vi "Modbus Status ES.vi"(0 "InterfaceData":T3 {"GenEast"."TotalFuel(L)" format="%.2f"; "GenEast"."FuelRate(L/H)" format="%.2f"; "GenEast"."ApparentPower(VA)" format="%.2f"; "GenEast"."BattVoltage(V)" format="%.2f"; "GenEast"."Freq(Hz)" format="%.2f"; "GenEast"."RunHours(hr)" format="%.2f"; "GenEast"."PowerFactor" format="%.2f"; "GenEast"."ReactivePower(VAR)" format="%.2f"; "GenEast"."ActivePower(W)" format="%.2f"; "GenWest"."TotalFuel(L)" format="%.2f"; "GenWest"."FuelRate(L/H)" format="%.2f"; "GenWest"."ApparentPower(VA)" format="%.2f"; "GenWest"."BattVoltage(V)" format="%.2f"; "GenWest"."Freq(Hz)" format="%.2f"; "GenWest"."RunHours(hr)" format="%.2f"; "GenWest"."PowerFactor" format="%.2f"; "GenWest"."ReactivePower(VAR)" format="%.2f"; "GenWest"."ActivePower(W)" format="%.2f"; "Converter Alarms 2" format="%016b"; "Converter Faults 2" format="%016b"; "Controller Faults" format="%016b"; "System Status" format="%016b"; "Converter Alarms 1" format="%016b"; "Converter Faults 1" format="%016b"; "Solar Faults" format="%016b"; "ES Rack 10 Alarms" format="%016b"; "ES Rack 9 Alarms" format="%016b"; "ES Rack 8 Alarms" format="%016b"; "ES Rack 7 Alarms" format="%016b"; "ES Rack 6 Alarms" format="%016b"; "ES Rack 5 Alarms" format="%016b"; "ES Rack 4 Alarms" format="%016b"; "ES Rack 3 Alarms" format="%016b"; "ES Rack 2 Alarms" format="%016b"; "ES Rack 1 Alarms" format="%016b"; "ES System Alarms" format="%016b"; "System Faults" format="%016b"; "ES Rack 10 Faults" format="%016b"; "ES Rack 9 Faults" format="%016b"; "ES Rack 8 Faults" format="%016b"; "ES Rack 7  Faults" format="%016b"; "ES Rack 6 Faults" format="%016b"; "ES Rack 5 Faults" format="%016b"; "ES Rack 4 Faults" format="%016b"; "ES Rack 3 Faults" format="%016b"; "ES Rack 2 Faults" format="%016b"; "ES Rack 1 Faults" format="%016b"; "ES System Faults" format="%016b"}, 1 "ES Cycle Count":dbl, 5 "ES String Data":T1, 9 "ES System Data In":T5={"Voltage"=0.0, "Current"=0.0, "SOC Avg"=0.0, "Faults"=0, "Alarms"=0, "# Strings"=0, "Max Temp"=0, "Min Temp"=0, "Max Cell Voltage"=0.0, "Min Cell Voltage"=0.0, "Energy Capacity"=0.0, "Energy Remaining"=0.0, "SOC Min"=0.0, "SOC Max"=0.0, "ES Fault"=FALSE, "String Select"=enum."3 Strings", "ES Com Fault"=FALSE, "SOH Avg"=0.0}, 11 "Error In":errorcluster) -> (4 "InterfaceData":T3 {"GenEast"."TotalFuel(L)" format="%.2f"; "GenEast"."FuelRate(L/H)" format="%.2f"; "GenEast"."ApparentPower(VA)" format="%.2f"; "GenEast"."BattVoltage(V)" format="%.2f"; "GenEast"."Freq(Hz)" format="%.2f"; "GenEast"."RunHours(hr)" format="%.2f"; "GenEast"."PowerFactor" format="%.2f"; "GenEast"."ReactivePower(VAR)" format="%.2f"; "GenEast"."ActivePower(W)" format="%.2f"; "GenWest"."TotalFuel(L)" format="%.2f"; "GenWest"."FuelRate(L/H)" format="%.2f"; "GenWest"."ApparentPower(VA)" format="%.2f"; "GenWest"."BattVoltage(V)" format="%.2f"; "GenWest"."Freq(Hz)" format="%.2f"; "GenWest"."RunHours(hr)" format="%.2f"; "GenWest"."PowerFactor" format="%.2f"; "GenWest"."ReactivePower(VAR)" format="%.2f"; "GenWest"."ActivePower(W)" format="%.2f"; "Converter Alarms 2" format="%016b"; "Converter Faults 2" format="%016b"; "Controller Faults" format="%016b"; "System Status" format="%016b"; "Converter Alarms 1" format="%016b"; "Converter Faults 1" format="%016b"; "Solar Faults" format="%016b"; "ES Rack 10 Alarms" format="%016b"; "ES Rack 9 Alarms" format="%016b"; "ES Rack 8 Alarms" format="%016b"; "ES Rack 7 Alarms" format="%016b"; "ES Rack 6 Alarms" format="%016b"; "ES Rack 5 Alarms" format="%016b"; "ES Rack 4 Alarms" format="%016b"; "ES Rack 3 Alarms" format="%016b"; "ES Rack 2 Alarms" format="%016b"; "ES Rack 1 Alarms" format="%016b"; "ES System Alarms" format="%016b"; "System Faults" format="%016b"; "ES Rack 10 Faults" format="%016b"; "ES Rack 9 Faults" format="%016b"; "ES Rack 8 Faults" format="%016b"; "ES Rack 7  Faults" format="%016b"; "ES Rack 6 Faults" format="%016b"; "ES Rack 5 Faults" format="%016b"; "ES Rack 4 Faults" format="%016b"; "ES Rack 3 Faults" format="%016b"; "ES Rack 2 Faults" format="%016b"; "ES Rack 1 Faults" format="%016b"; "ES System Faults" format="%016b"}, 15 "Error Out":errorcluster)   [LabVIEW 2014]
uses:
  Controls/ES System Data.ctl
  Controls/StringSelector.ctl
  Controls/Interface Data.ctl
  Controls/Gen Data.ctl
  Controls/ES String Array.ctl
  Controls/ES String Data.ctl
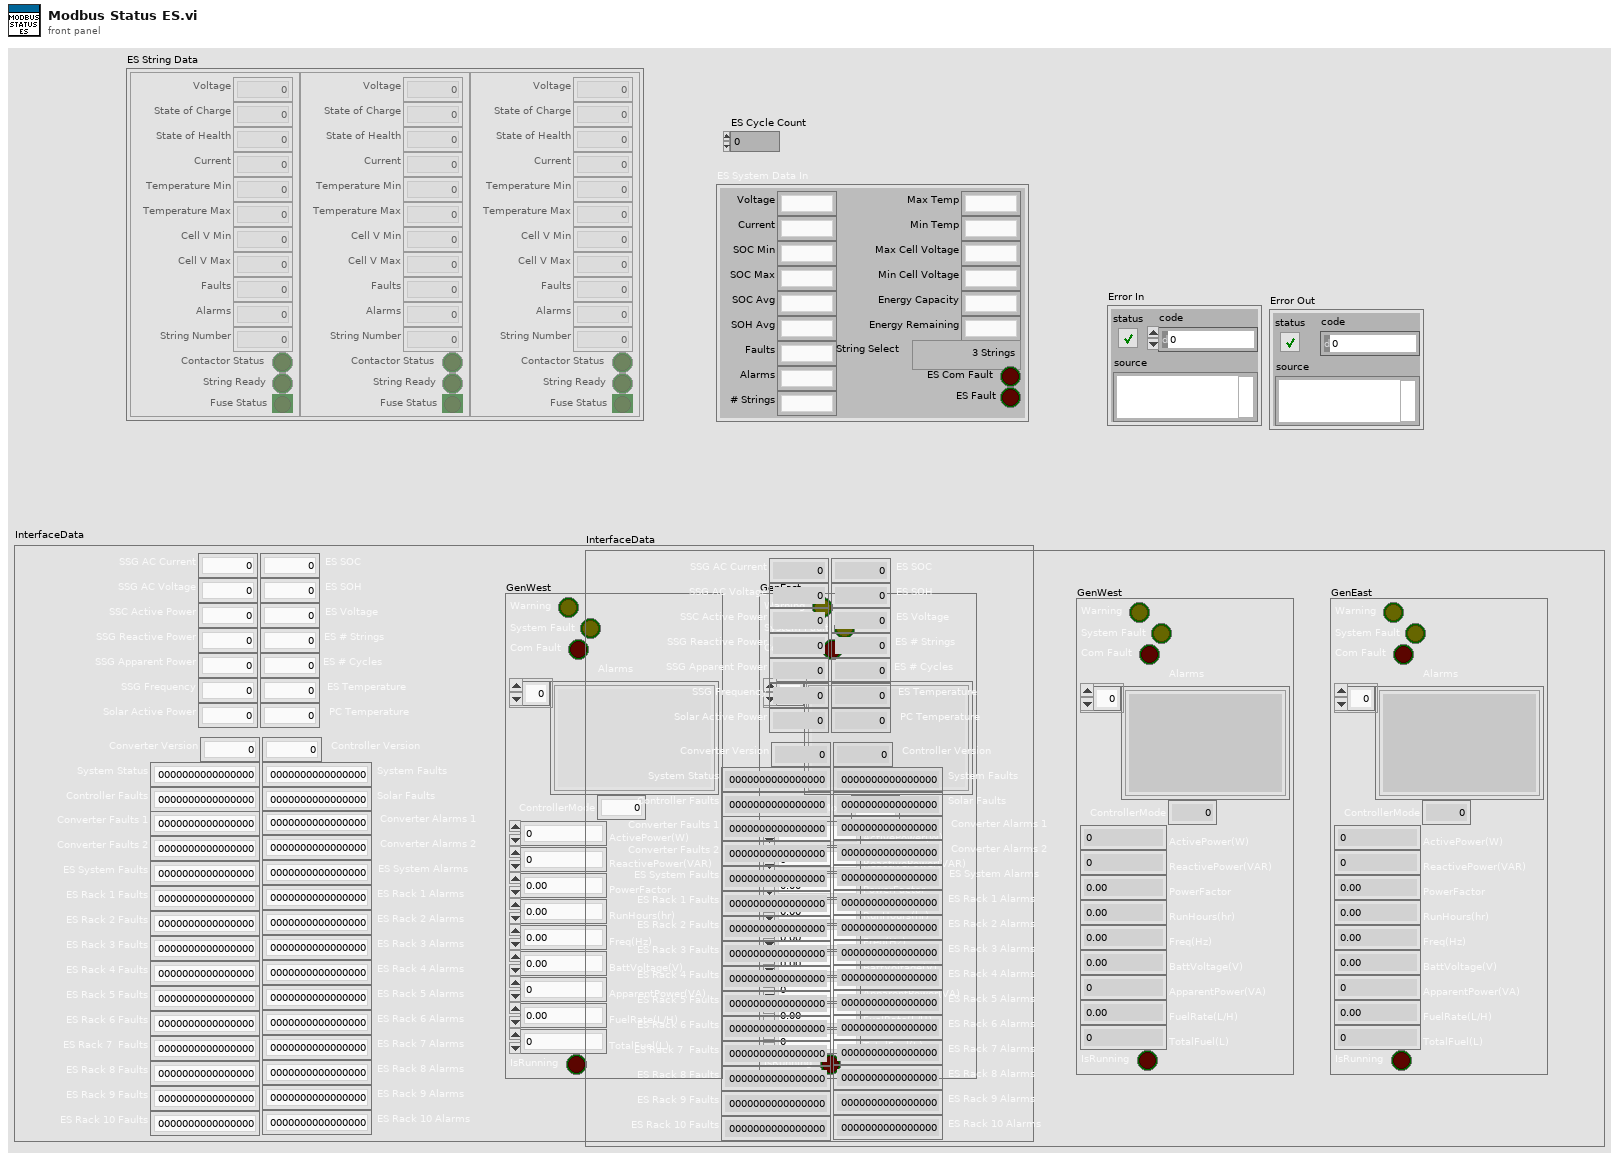
[diagram p1: front panel]
types:
  T1 = typedef "ES String Array.ctl" = T2[]
  T2 = typedef "ES String Data.ctl" = cluster{"Voltage":sgl, "State of Charge":sgl, "Current":sgl, "Temperature Min":i16, "Temperature Max":i16, "Faults":u16, "Alarms":u16, "String Number":u16, "Contactor Status":bool, "String Ready":bool, "Fuse Status":bool, "Cell V Max":dbl, "Cell V Min":dbl, "State of Health":sgl}
  T3 = typedef "Interface Data.ctl" = cluster{"SSG AC Current":i16, "SSG AC Voltage":i16, "SSC Active Power":i16, "SSG Reactive Power":i16, "SSG Apparent Power":i16, "SSG Frequency":i16, "ES SOC":i16, "ES SOH":i16, "ES Voltage":i16, "ES # Strings":i16, "ES # Cycles":i16, "ES Temperature":i16, "PC Temperature":i16, "Solar Active Power":i16, "Converter Version":i16, "Controller Version":i16, "System Status":i16, "System Faults":i16, "Controller Faults":i16, "ES System Faults":i16, "ES System Alarms":i16, "Converter Faults 1":i16, "Converter Faults 2":i16, "Converter Alarms 1":i16, "Converter Alarms 2":i16, "Solar Faults":i16, "ES Rack 1 Faults":i16, "ES Rack 2 Faults":i16, "ES Rack 3 Faults":i16, "ES Rack 4 Faults":i16, "ES Rack 5 Faults":i16, "ES Rack 6 Faults":i16, "ES Rack 7  Faults":i16, "ES Rack 8 Faults":i16, "ES Rack 9 Faults":i16, "ES Rack 10 Faults":i16, "ES Rack 1 Alarms":i16, "ES Rack 2 Alarms":i16, "ES Rack 3 Alarms":i16, "ES Rack 4 Alarms":i16, "ES Rack 5 Alarms":i16, "ES Rack 6 Alarms":i16, "ES Rack 7 Alarms":i16, "ES Rack 8 Alarms":i16, "ES Rack 9 Alarms":i16, "ES Rack 10 Alarms":i16, "GenWest":T4, "GenEast":T4}
  T4 = typedef "Gen Data.ctl" = cluster{"Warning":bool, "System Fault":bool, "Com Fault":bool, "Alarms":string[], "ControllerMode":u16, "ActivePower(W)":i32, "ReactivePower(VAR)":i32, "PowerFactor":dbl, "RunHours(hr)":dbl, "Freq(Hz)":dbl, "BattVoltage(V)":dbl, "ApparentPower(VA)":i32, "FuelRate(L/H)":dbl, "TotalFuel(L)":u32, "IsRunning":bool}
  T5 = typedef "ES System Data.ctl" = cluster{"Voltage":sgl, "Current":sgl, "SOC Avg":sgl, "Faults":u16, "Alarms":u16, "# Strings":u16, "Max Temp":i16, "Min Temp":i16, "Max Cell Voltage":sgl, "Min Cell Voltage":sgl, "Energy Capacity":sgl, "Energy Remaining":sgl, "SOC Min":sgl, "SOC Max":sgl, "ES Fault":bool, "String Select":T6, "ES Com Fault":bool, "SOH Avg":sgl}
  T6 = typedef "StringSelector.ctl" = enum16{"1 String (1)", "1 String (2)", "1 String (3)", "2 Strings (1 2)", "2 Strings (2 3)", "2 Strings (1 3)", "3 Strings"}
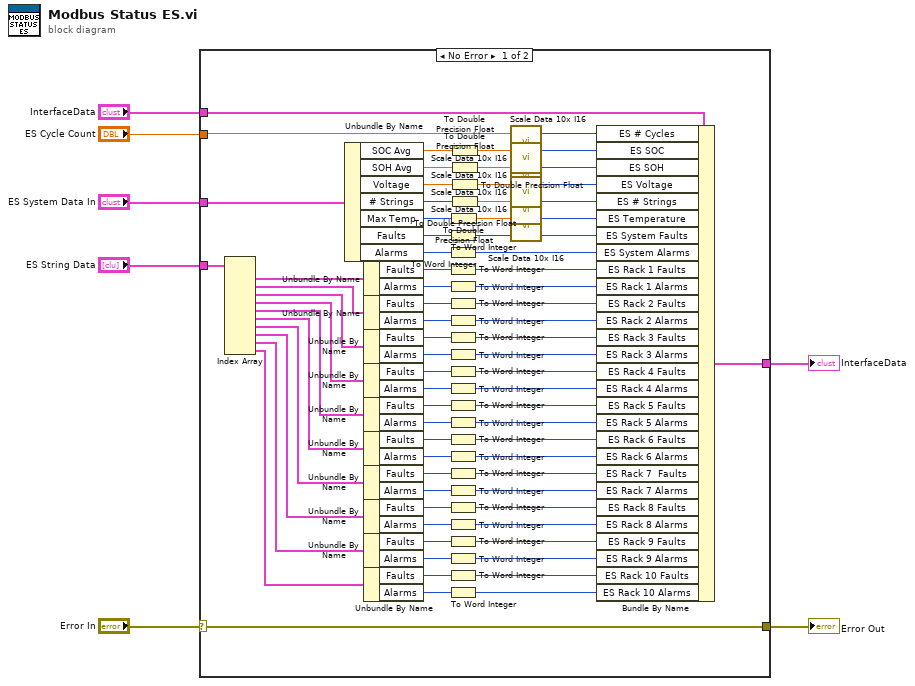
[diagram p0: block diagram]
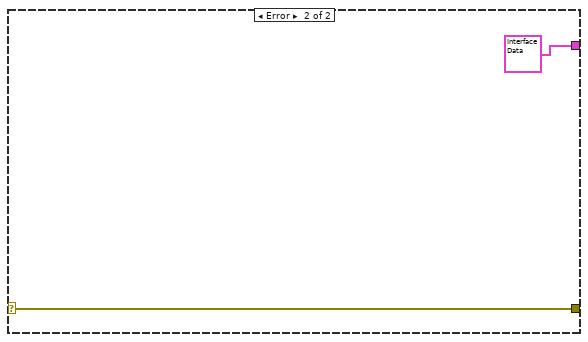
[diagram p2: hidden frame]
diagram:
  n1 = case shown="No Error" "Error In" {
    selector: "Error In" -> [w83 w84]
    tunnel: [w83 w84] -> w6
    tunnel: "ES System Data In" -> [w80 _]
    tunnel: "InterfaceData" -> [w82 _]
    tunnel: "ES String Data" -> [w60 _]
    tunnel: [w81 T3 {"SSG AC Current"=0, "SSG AC Voltage"=0, "SSC Active Power"=0, "SSG Reactive Power"=0, "SSG Apparent Power"=0, "SSG Frequency"=0, "ES SOC"=0, "ES SOH"=0, "ES Voltage"=0, "ES # Strings"=0, "ES # Cycles"=0, "ES Temperature"=0, "PC Temperature"=0, "Solar Active Power"=0, "Converter Version"=0, "Controller Version"=0, "System Status"=0, "System Faults"=0, "Controller Faults"=0, "ES System Faults"=0, "ES System Alarms"=0, "Converter Faults 1"=0, "Converter Faults 2"=0, "Converter Alarms 1"=0, "Converter Alarms 2"=0, "Solar Faults"=0, "ES Rack 1 Faults"=0, "ES Rack 2 Faults"=0, "ES Rack 3 Faults"=0, "ES Rack 4 Faults"=0, "ES Rack 5 Faults"=0, "ES Rack 6 Faults"=0, "ES Rack 7  Faults"=0, "ES Rack 8 Faults"=0, "ES Rack 9 Faults"=0, "ES Rack 10 Faults"=0, "ES Rack 1 Alarms"=0, "ES Rack 2 Alarms"=0, "ES Rack 3 Alarms"=0, "ES Rack 4 Alarms"=0, "ES Rack 5 Alarms"=0, "ES Rack 6 Alarms"=0, "ES Rack 7 Alarms"=0, "ES Rack 8 Alarms"=0, "ES Rack 9 Alarms"=0, "ES Rack 10 Alarms"=0, "GenWest"={"Warning"=FALSE, "System Fault"=FALSE, "Com Fault"=FALSE, "Alarms"=[], "ControllerMode"=0, "ActivePower(W)"=0, "ReactivePower(VAR)"=0, "PowerFactor"=0.0, "RunHours(hr)"=0.0, "Freq(Hz)"=0.0, "BattVoltage(V)"=0.0, "ApparentPower(VA)"=0, "FuelRate(L/H)"=0.0, "TotalFuel(L)"=0, "IsRunning"=FALSE}, "GenEast"={"Warning"=FALSE, "System Fault"=FALSE, "Com Fault"=FALSE, "Alarms"=[], "ControllerMode"=0, "ActivePower(W)"=0, "ReactivePower(VAR)"=0, "PowerFactor"=0.0, "RunHours(hr)"=0.0, "Freq(Hz)"=0.0, "BattVoltage(V)"=0.0, "ApparentPower(VA)"=0, "FuelRate(L/H)"=0.0, "TotalFuel(L)"=0, "IsRunning"=FALSE}} ("Modbus Status Interface Data Out")] -> w2
    tunnel: "ES Cycle Count" -> [w9 _]
    frame No Error {
      n2 = Index Array(array=w60) -> (element #1=w59:T2, element #2=w58:T2, element #3=w57:T2, element #4=w56:T2, element #5=w55:T2, element #6=w54:T2, element #7=w53:T2, element #8=w52:T2, element #9=w51:T2, element #10=w50:T2)  [unwired: 10 in]
      n3 = Unbundle By Name(w80) -> ("SOC Avg"=w78:sgl, "SOH Avg"=w76:sgl, "Voltage"=w74:sgl, "# Strings"=w72:u16, "Max Temp"=w70:i16, "Faults"=w64:u16, "Alarms"=w63:u16)
      n4 = Unbundle By Name(w59) -> ("Faults"=w49:u16, "Alarms"=w48:u16)
      n5 = Unbundle By Name(w58) -> ("Faults"=w47:u16, "Alarms"=w46:u16)
      n6 = Unbundle By Name(w57) -> ("Faults"=w45:u16, "Alarms"=w44:u16)
      n7 = Unbundle By Name(w56) -> ("Faults"=w43:u16, "Alarms"=w42:u16)
      n8 = Unbundle By Name(w55) -> ("Faults"=w41:u16, "Alarms"=w40:u16)
      n9 = Unbundle By Name(w54) -> ("Faults"=w39:u16, "Alarms"=w38:u16)
      n10 = Unbundle By Name(w53) -> ("Faults"=w37:u16, "Alarms"=w36:u16)
      n11 = Unbundle By Name(w52) -> ("Faults"=w35:u16, "Alarms"=w34:u16)
      n12 = Unbundle By Name(w51) -> ("Faults"=w33:u16, "Alarms"=w32:u16)
      n13 = Unbundle By Name(w50) -> ("Faults"=w31:u16, "Alarms"=w30:u16)
      n14 = To Word Integer(number=w64) -> (16bit integer=w62:i16)
      n15 = To Word Integer(number=w63) -> (16bit integer=w61:i16)
      n16 = To Word Integer(number=w49) -> (16bit integer=w29:i16)
      n17 = To Word Integer(number=w48) -> (16bit integer=w28:i16)
      n18 = To Word Integer(number=w47) -> (16bit integer=w27:i16)
      n19 = To Word Integer(number=w46) -> (16bit integer=w26:i16)
      n20 = To Word Integer(number=w45) -> (16bit integer=w25:i16)
      n21 = To Word Integer(number=w44) -> (16bit integer=w24:i16)
      n22 = To Word Integer(number=w43) -> (16bit integer=w23:i16)
      n23 = To Word Integer(number=w42) -> (16bit integer=w22:i16)
      n24 = To Word Integer(number=w41) -> (16bit integer=w21:i16)
      n25 = To Word Integer(number=w40) -> (16bit integer=w20:i16)
      n26 = To Word Integer(number=w39) -> (16bit integer=w19:i16)
      n27 = To Word Integer(number=w38) -> (16bit integer=w18:i16)
      n28 = To Word Integer(number=w37) -> (16bit integer=w17:i16)
      n29 = To Word Integer(number=w36) -> (16bit integer=w16:i16)
      n30 = To Word Integer(number=w35) -> (16bit integer=w15:i16)
      n31 = To Word Integer(number=w34) -> (16bit integer=w14:i16)
      n32 = To Word Integer(number=w33) -> (16bit integer=w13:i16)
      n33 = To Word Integer(number=w32) -> (16bit integer=w12:i16)
      n34 = To Word Integer(number=w31) -> (16bit integer=w11:i16)
      n35 = To Word Integer(number=w30) -> (16bit integer=w10:i16)
      n36 = To Double Precision Float(number=w70) -> (double precision float=w65:dbl)
      n37 = To Double Precision Float(number=w78) -> (double precision float=w77:dbl)
      n38 = To Double Precision Float(number=w76) -> (double precision float=w66:dbl)
      n39 = To Double Precision Float(number=w74) -> (double precision float=w67:dbl)
      n40 = To Double Precision Float(number=w72) -> (double precision float=w68:dbl)
      n41 = call "Scale Data 10x I16.vi"("Data In"=w9) -> ("16bit integer"=w8:i16)  [unwired: 2 in]
      n42 = call "Scale Data 10x I16.vi"("Data In"=w77) -> ("16bit integer"=w79:i16)  [unwired: 2 in]
      n43 = call "Scale Data 10x I16.vi"("Data In"=w66) -> ("16bit integer"=w75:i16)  [unwired: 2 in]
      n44 = call "Scale Data 10x I16.vi"("Data In"=w67) -> ("16bit integer"=w73:i16)  [unwired: 2 in]
      n45 = call "Scale Data 10x I16.vi"("Data In"=w68) -> ("16bit integer"=w71:i16)  [unwired: 2 in]
      n46 = call "Scale Data 10x I16.vi"("Data In"=w65) -> ("16bit integer"=w69:i16)  [unwired: 2 in]
      n47 = Bundle By Name(cluster=w82, "ES # Cycles"=w8, "ES SOC"=w79, "ES SOH"=w75, "ES Voltage"=w73, "ES # Strings"=w71, "ES Temperature"=w69, "ES System Faults"=w62, "ES System Alarms"=w61, "ES Rack 1 Faults"=w29, "ES Rack 1 Alarms"=w28, "ES Rack 2 Faults"=w27, "ES Rack 2 Alarms"=w26, "ES Rack 3 Faults"=w25, "ES Rack 3 Alarms"=w24, "ES Rack 4 Faults"=w23, "ES Rack 4 Alarms"=w22, "ES Rack 5 Faults"=w21, "ES Rack 5 Alarms"=w20, "ES Rack 6 Faults"=w19, "ES Rack 6 Alarms"=w18, "ES Rack 7  Faults"=w17, "ES Rack 7 Alarms"=w16, "ES Rack 8 Faults"=w15, "ES Rack 8 Alarms"=w14, "ES Rack 9 Faults"=w13, "ES Rack 9 Alarms"=w12, "ES Rack 10 Faults"=w11, "ES Rack 10 Alarms"=w10) -> (w81:T3)
    }
    frame Error {
    }
  }
  "Error Out" <- w6
  "InterfaceData" <- w2
